vi "GEOM_FindMaximunAmountOfAlignedAmps.vi"(9 "how":enum16{"rows (y)", "columns (x)"}(ring), 10 "amplifiers":T1[](array[typedef]) {"fliped" items=["none", "horizontal", "vertical"]; "type" items=["LL", "LR", "UL", "UR"]}) -> (1 "maxalignedamps":i32, 2 "max":i32)   [LabVIEW 2016]
uses:
  GEOM_Amplifier.ctl
  GEOM_AmpType.ctl
  GEOM_ROI.ctl
  GEOM_Coords.ctl
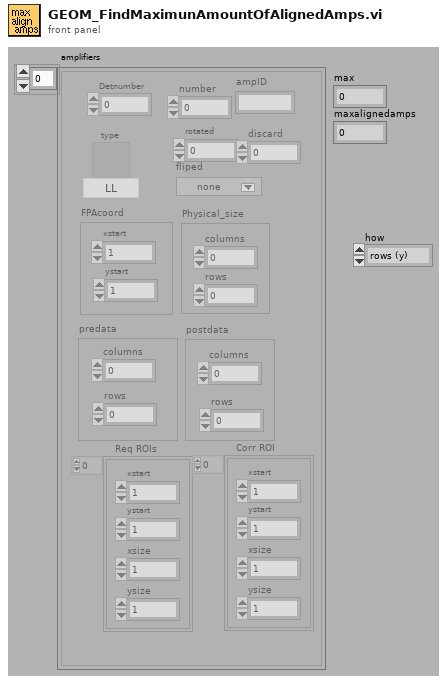
[diagram p1: front panel]
types:
  T1 = typedef "GEOM_Amplifier.ctl" = cluster{"number":i32, "type":T2, "rotated":i16, "fliped":u16, "FPAcoord":cluster{"xstart":i32, "ystart":i32}, "Physical_size":cluster{"columns":i32, "rows":i32}, "predata":cluster{"columns":i32, "rows":i32}, "postdata":cluster{"columns":i32, "rows":i32}, "Req ROIs":T3, "Corr ROI":T3, "Detnumber":i32, "ampID":string, "discard":i32}
  T2 = typedef "GEOM_AmpType.ctl" = u16
  T3 = typedef "GEOM_ROI.ctl" = T4[]
  T4 = typedef "GEOM_Coords.ctl" = cluster{"xstart":u32, "ystart":u32, "xsize":u32, "ysize":u32}
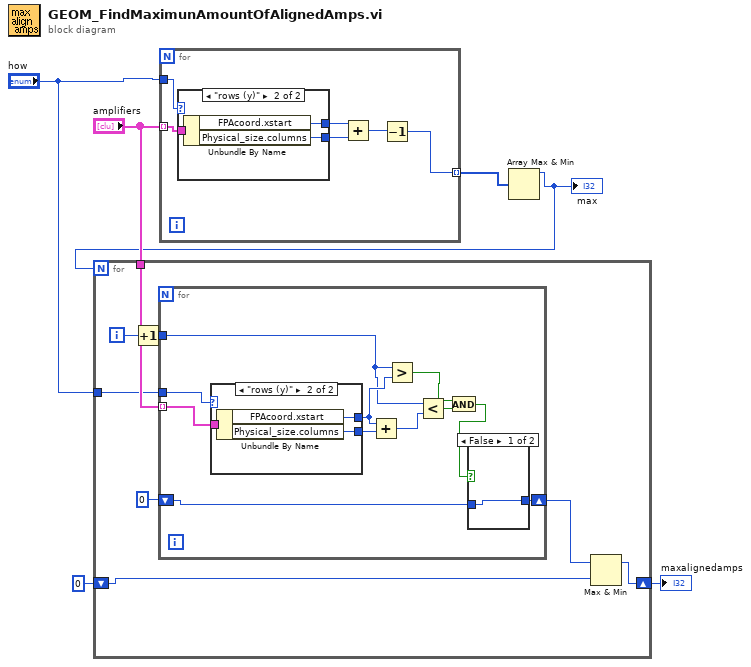
[diagram p0: block diagram]
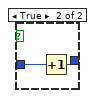
[diagram p2: hidden frame]
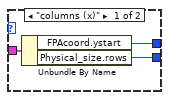
[diagram p3: hidden frame]
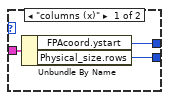
[diagram p4: hidden frame]
diagram:
  n1 = for {
    tunnel: "amplifiers" -> [w12] mode=indexing
    tunnel: [w8] -> w6 mode=indexing
    tunnel: "how" -> [w7]
    n2 = case shown="\"rows (y)\"" w7 {
      tunnel: w12 -> [w15 w18]
      tunnel: [w14 w17] -> w11
      tunnel: [w13 w16] -> w10
      frame "columns (x)" {
        n3 = Unbundle By Name(w15) -> ("FPAcoord.ystart"=w14:i32, "Physical_size.rows"=w13:i32)
      }
      frame "rows (y)" {
        n4 = Unbundle By Name(w18) -> ("FPAcoord.xstart"=w17:i32, "Physical_size.columns"=w16:i32)
      }
    }
    n5 = Add(x=w11, y=w10) -> (x+y=w9:i32)
    n6 = Decrement(x=w9) -> (x-1=w8:i32)
  }
  n7 = Array Max & Min(array=w6) -> (max value=w3:i32)  [unwired: 3 out]
  "max" <- w3
  n8 = for {
    N: w3 -> [_]
    tunnel: "amplifiers" -> [w26]
    tunnel: "how" -> [w25]
    shift-right: [w20] -> w2
    shift-left: 0 -> [w19]
    i -> [w24]
    n9 = Increment(x=w24) -> (x+1=w23:i32)
    n10 = for {
      tunnel: w26 -> [w37] mode=indexing
      tunnel: w25 -> [w36]
      tunnel: w23 -> [w31]
      shift-right: [w27] -> w21
      shift-left: 0 -> [w28]
      n11 = case shown="\"rows (y)\"" w36 {
        tunnel: w37 -> [w43 w46]
        tunnel: [w42 w45] -> w32
        tunnel: [w41 w44] -> w35
        frame "columns (x)" {
          n12 = Unbundle By Name(w43) -> ("FPAcoord.ystart"=w42:i32, "Physical_size.rows"=w41:i32)
        }
        frame "rows (y)" {
          n13 = Unbundle By Name(w46) -> ("FPAcoord.xstart"=w45:i32, "Physical_size.columns"=w44:i32)
        }
      }
      n14 = Add(x=w32, y=w35) -> (x+y=w30:i32)
      n15 = Greater?(x=w31, y=w32) -> (0:w33:bool)
      n16 = Less?(x=w31, y=w30) -> (x < y?=w34:bool)
      n17 = And(x=w33, y=w34) -> (x .and. y?=w29:bool)
      n18 = case shown="False" w29 {
        tunnel: w28 -> [w38 w40]
        tunnel: [w38 w39] -> w27
        frame False {
        }
        frame True {
          n19 = Increment(x=w40) -> (x+1=w39:i32)
        }
      }
    }
    n20 = Max & Min(x=w21, y=w19) -> (max(x,y)=w20:i32)  [unwired: 1 out]
  }
  "maxalignedamps" <- w2
